vi "Remove all sections.vi"(11 "info data":string) -> (3 "info data out":string)   [LabVIEW 2019, in "infolib.lvlib"]
doc: "Remove all sections and returns the rest. Contain infinite loop, but every iteration something should be removed, so the loop should always end."
uses:
  infolib.lvlib
  <vilib>/regexp/Match Regular Expression.xnode
panel:
  # "testing string:"
  # "test1\ntest2\n#startsection:: 1\nAAA\n#startsection:: 2\nBBB\n\t  \t#endsection:: 2\nCCC\n#endsection:: 1\ntest3\ntest4\n#startsection:: X\nDDD\n#endsection:: X\ntest5"
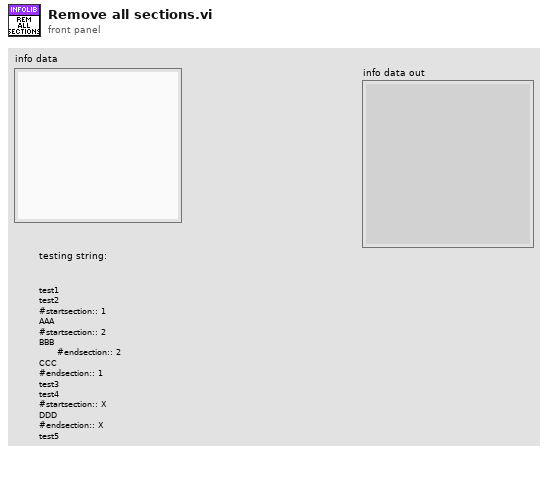
[diagram p1: front panel]
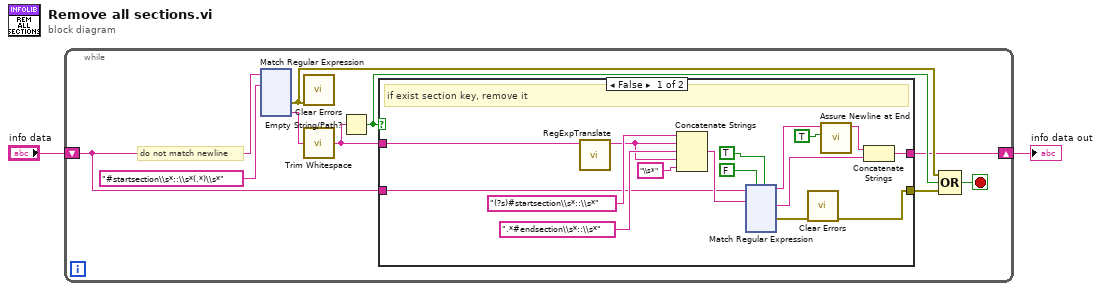
[diagram p0: block diagram]
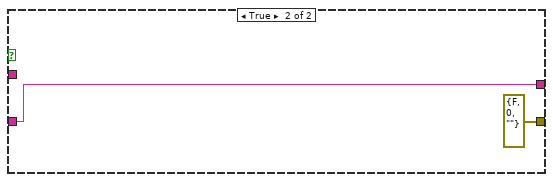
[diagram p2: hidden frame]
diagram:
  n1 = while {
    shift-right: [w4] -> w1
    shift-left: "info data" -> [w5]
    stop <- w11 stop-if-true
    # "do not match newline"
    n2 = xnode "Match Regular Expression"("input string"=w5, "regular expression"="#startsection\\s*::\\s*(.*)\\s*" ("section name")) -> ("error out"=w9:errorcluster, "submatch 1"=w8:string)  [unwired: 4 in, 4 out]
    n3 = call <vilib>:"Clear Errors.vi"("error in (no error)"=w9) -> ()  [unwired: 5 in, 2 out]
    n4 = call <vilib>:"Trim Whitespace.vi"("string"=w8) -> ("trimmed string"=w6:string)  [unwired: 1 in]
    n5 = Empty String/Path?(string/path=w6) -> (empty?=w7:bool)
    n6 = case shown="False" w7 {
      tunnel: w6 -> [w13 _]
      tunnel: w5 -> [w21 w145]
      tunnel: [w17 w145] -> w4
      tunnel: [w15 errorcluster {"status"=FALSE, "code"=0, "source"=""} ("error out")] -> w3
      frame False {
        # "if exist section key, remove it"
        n7 = call "RegExpTranslate.vi"("string"=w13) -> ("regexp safe string"=w12:string)  [unwired: 10 in]
        n8 = Concatenate Strings("(?s)#startsection\\s*::\\s*" ("section name"), w12, ".*#endsection\\s*::\\s*" ("section name"), w12, "\\s*" ("section name")) -> (w22:string)
        n9 = xnode "Match Regular Expression"("input string"=w21, "regular expression"=w22, "ignore case? (F)"=FALSE, "multiline? (F)"=TRUE) -> ("before match"=w20:string, "after match"=w18:string, "error out"=w16:errorcluster)  [unwired: 2 in, 3 out]
        n10 = call <vilib>:"Clear Errors.vi"("error in (no error)"=w16) -> ("error out"=w15:errorcluster)  [unwired: 5 in, 1 out]
        n11 = call "Assure Newline at End.vi"("Set End Of Line (F)"=TRUE, "string"=w20) -> ("string out"=w19:string)  [unwired: 9 in]
        n12 = Concatenate Strings(w19, w18) -> (w17:string)
      }
      frame True {
      }
    }
    n13 = Compound Arithmetic op=OR(w9, w7, w3) -> (w11:bool)
  }
  "info data out" <- w1
